vi "Disable_Enable.vi"(6 "menu reference":refnum<k9>, 7 "Disabled":T2(ring)=enum."Disabled and Grayed Out", 8 "error in (no error)":errorcluster, 10 "Command":T1=enum."INIT", 11 "EpiWrapper in":refnum<class "EpiWrapper.lvclass">) -> (0 "error out":errorcluster, 3 "EpiWrapper out":refnum<class "EpiWrapper.lvclass">)   [LabVIEW 2012, in "EpiWrapper.lvclass"]
uses:
  EpiWrapper.lvclass
  Controls/Command_Enum.ctl
  Controls/Control_Selector.ctl
  Controls/Input_Selector.ctl
  EpiWrapper.lvclass/EpiWrapper.ctl
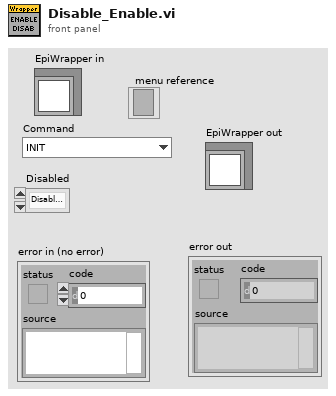
[diagram p1: front panel]
types:
  T1 = typedef "Command_Enum.ctl" = enum16{"SPECTRUMCAPTURE", "INSITUMEASURE", "RESETCONFIG", "OPENCONFIG", "RESET", "INIT", "LOAD", "MEASURE", "NEW", "SAVE", "UPDATE_INT", "SWAP_MODE", "UPDATE_ACQ", "MARK_MAP_SELECT", "MARK_MAP", "EXIT", "CANCEL"}
  T2 = enum8{"Enabled", "Disabled", "Disabled and Grayed Out"}
  T3 = typedef "Input_Selector.ctl" = enum16{"Wafer ID", "Test", "New", "Save", "Load", "Cancel"}
  T4 = typedef "Control_Selector.ctl" = enum16{"Plot", "Pass", "Fail", "Measure", "Area", "TestData", "Pad"}
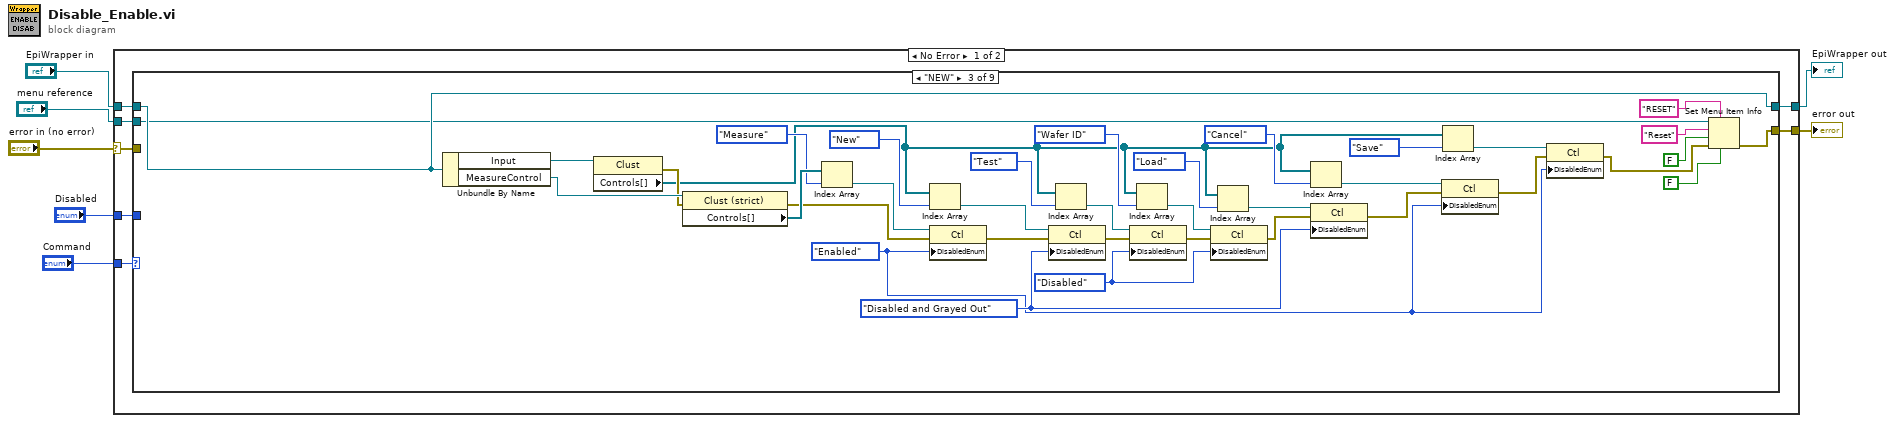
[diagram p0: block diagram]
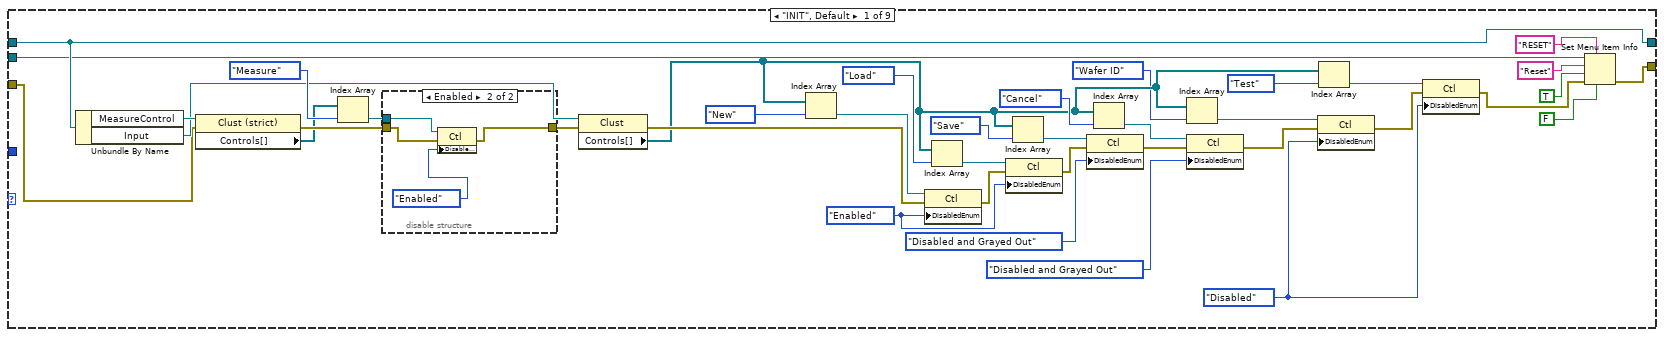
[diagram p2: hidden frame]
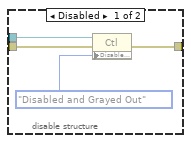
[diagram p3: hidden frame]
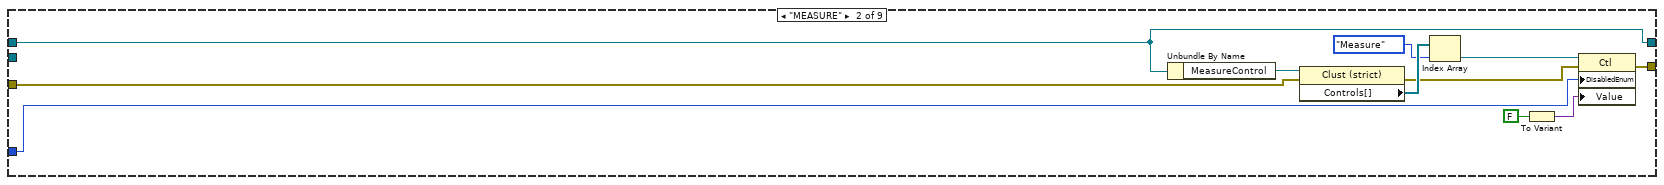
[diagram p4: hidden frame]
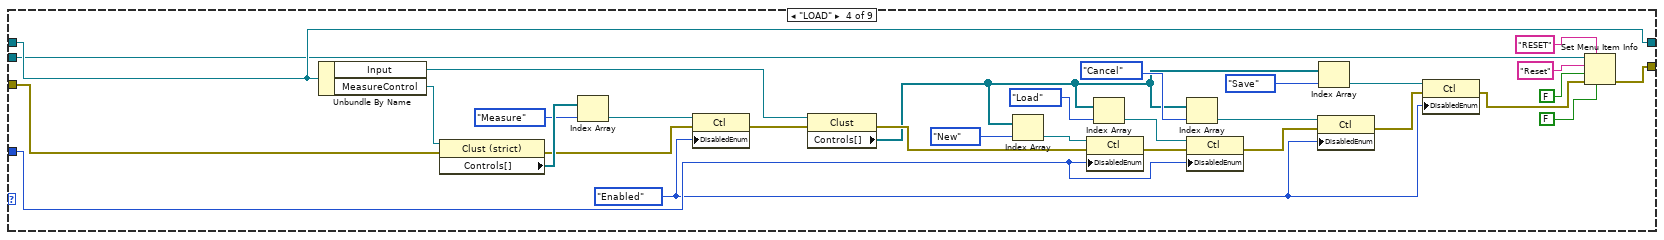
[diagram p5: hidden frame]
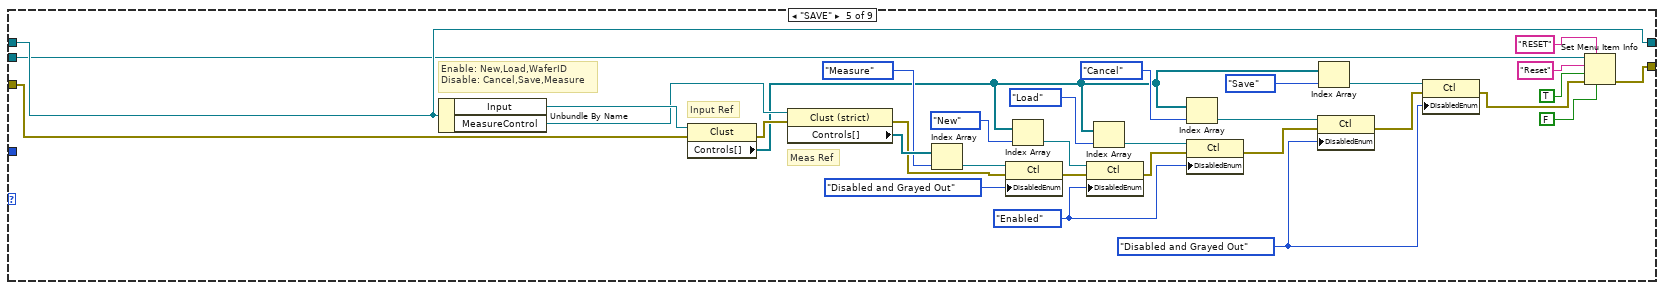
[diagram p6: hidden frame]
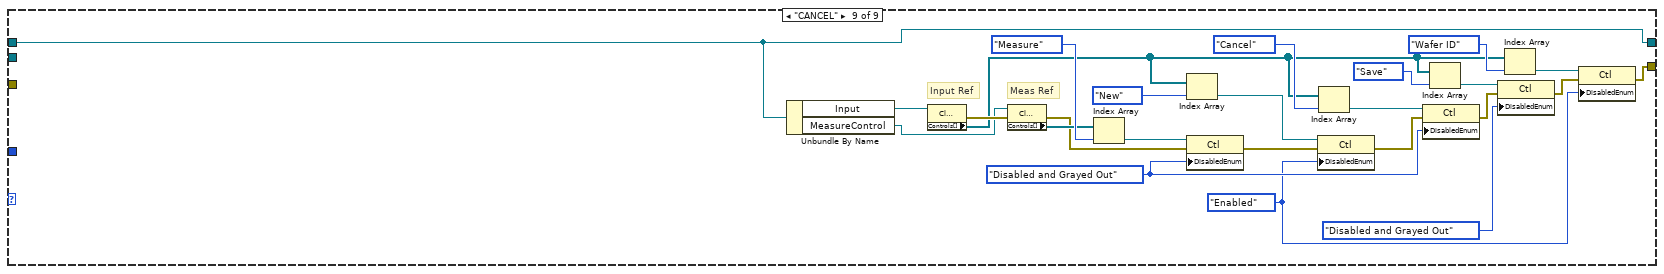
[diagram p10: hidden frame]
diagram:
  n1 = case shown="No Error" "error in (no error)" {
    selector: "error in (no error)" -> [w10 w205]
    tunnel: [w11 w205] -> w6
    tunnel: [w9 w204] -> w4
    tunnel: "EpiWrapper in" -> [w13 w204]
    tunnel: "Command" -> [w14 _]
    tunnel: "Disabled" -> [w12 _]
    tunnel: "menu reference" -> [w8 _]
    frame No Error {
      n2 = case shown="\"NEW\"" w14 {
        tunnel: w13 -> [w44 w64 w96 w132 w154 w174 w176 w178 w191]
        tunnel: w12 -> [_ w65 _ w135 _ _ _ _ _]
        tunnel: [w17 w66 w73 w112 w147 w173 w175 w177 w179] -> w11
        tunnel: w10 -> [w15 w68 _ w130 w153 w173 w175 w177 _]
        tunnel: [w44 w64 w96 w132 w154 w174 w176 w178 w191] -> w9
        tunnel: w8 -> [w16 _ w75 w110 w145 _ _ _ _]
        frame "INIT", Default {
          w23 = T2."Disabled" ("Disabled")
          w33 = T2."Enabled" ("Disabled")
          n3 = Unbundle By Name(w44) -> ("MeasureControl"=w47:refnum<vi>, "Input"=w46:refnum<vi>)
          n4 = property class="Clust (strict)"(reference=w47, error in=w15) -> (error out=w50:errorcluster, "Controls[]"=w45:refnum<vi>[])  [unwired: 1 out]
          n5 = Index Array(array=w45, index=Control_Selector."Measure" ("Control_Selector")) -> (element=w49:refnum<vi>)
          n6 = disable-structure shown="Enabled" {
            disable-tunnel: [w57 w59] -> w53
            disable-tunnel: w50 -> [w56 w60]
            disable-tunnel: w49 -> [w55 w61]
            frame Disabled {
              n7 = property class="Ctl"(reference=w55, error in=w56, "DisabledEnum"=T2."Disabled and Grayed Out" ("Disabled")) -> (error out=w57:errorcluster)  [unwired: 1 out]
            }
            frame Enabled {
              n8 = property class="Ctl"(reference=w61, error in=w60, "DisabledEnum"=T2."Enabled" ("Disabled")) -> (error out=w59:errorcluster)  [unwired: 1 out]
            }
          }
          n9 = property class="Clust"(reference=w46, error in=w53) -> (error out=w37:errorcluster, "Controls[]"=w30:refnum<vi>[])  [unwired: 1 out]
          n10 = Index Array(array=w30, index=Input_Selector."New" ("InputSelector")) -> (element=w51:refnum<vi>)
          n11 = property class="Ctl"(reference=w51, error in=w37, "DisabledEnum"=w33) -> (error out=w32:errorcluster)  [unwired: 1 out]
          n12 = Index Array(array=w30, index=Input_Selector."Load" ("InputSelector")) -> (element=w34:refnum<vi>)
          n13 = property class="Ctl"(reference=w34, error in=w32, "DisabledEnum"=w33) -> (error out=w31:errorcluster)  [unwired: 1 out]
          n14 = Index Array(array=w30, index=Input_Selector."Save" ("InputSelector")) -> (element=w39:refnum<vi>)
          n15 = property class="Ctl"(reference=w39, error in=w31, "DisabledEnum"=T2."Disabled and Grayed Out" ("Disabled")) -> (error out=w36:errorcluster)  [unwired: 1 out]
          n16 = Index Array(array=w30, index=Input_Selector."Cancel" ("InputSelector")) -> (element=w38:refnum<vi>)
          n17 = Index Array(array=w30, index=Input_Selector."Wafer ID" ("InputSelector")) -> (element=w25:refnum<vi>)
          n18 = property class="Ctl"(reference=w38, error in=w36, "DisabledEnum"=T2."Disabled and Grayed Out" ("Disabled")) -> (error out=w26:errorcluster)  [unwired: 1 out]
          n19 = property class="Ctl"(reference=w25, error in=w26, "DisabledEnum"=w23) -> (error out=w27:errorcluster)  [unwired: 1 out]
          n20 = Index Array(array=w30, index=Input_Selector."Test" ("InputSelector")) -> (element=w24:refnum<vi>)
          n21 = property class="Ctl"(reference=w24, error in=w27, "DisabledEnum"=w23) -> (error out=w18:errorcluster)  [unwired: 1 out]
          n22 = Set Menu Item Info(6:FALSE ("checked"), 7:"RESET" ("item name"), 8:w18, 9:TRUE ("enabled"), 10:"Reset" ("item name"), 11:w16) -> (0:w17:errorcluster)  [unwired: 1 in, 1 out]
        }
        frame "MEASURE" {
          n23 = Unbundle By Name(w64) -> ("MeasureControl"=w71:refnum<vi>)
          n24 = property class="Clust (strict)"(reference=w71, error in=w68) -> (error out=w67:errorcluster, "Controls[]"=w72:refnum<vi>[])  [unwired: 1 out]
          n25 = Index Array(array=w72, index=Control_Selector."Measure" ("Control_Selector")) -> (element=w69:refnum<vi>)
          n26 = To Variant(anything=FALSE) -> (Variant=w62:variant)
          n27 = property class="Ctl"(reference=w69, error in=w67, "DisabledEnum"=w65, "Value"=w62) -> (error out=w66:errorcluster)  [unwired: 1 out]
        }
        frame "NEW" {
          w85 = T2."Disabled" ("Disabled")
          w88 = T2."Disabled and Grayed Out" ("Disabled")
          w81 = T2."Enabled" ("Disabled")
          n28 = Unbundle By Name(w96) -> ("Input"=w108:refnum<vi>, "MeasureControl"=w106:refnum<vi>)
          n29 = property class="Clust"(reference=w108) -> (error out=w105:errorcluster, "Controls[]"=w83:refnum<vi>[])  [unwired: 1 in, 1 out]
          n30 = property class="Clust (strict)"(reference=w106, error in=w105) -> (error out=w101:errorcluster, "Controls[]"=w104:refnum<vi>[])  [unwired: 1 out]
          n31 = Index Array(array=w104, index=Control_Selector."Measure" ("Control_Selector")) -> (element=w102:refnum<vi>)
          n32 = Index Array(array=w83, index=Input_Selector."New" ("InputSelector")) -> (element=w109:refnum<vi>)
          n33 = property class="Ctl"(reference=w102, error in=w101, "DisabledEnum"=w81) -> (error out=w100:errorcluster)  [unwired: 1 out]
          n34 = property class="Ctl"(reference=w109, error in=w100, "DisabledEnum"=w88) -> (error out=w93:errorcluster)  [unwired: 1 out]
          n35 = Index Array(array=w83, index=Input_Selector."Test" ("InputSelector")) -> (element=w94:refnum<vi>)
          n36 = property class="Ctl"(reference=w94, error in=w93, "DisabledEnum"=w85) -> (error out=w92:errorcluster)  [unwired: 1 out]
          n37 = Index Array(array=w83, index=Input_Selector."Wafer ID" ("InputSelector")) -> (element=w98:refnum<vi>)
          n38 = property class="Ctl"(reference=w98, error in=w92, "DisabledEnum"=w85) -> (error out=w89:errorcluster)  [unwired: 1 out]
          n39 = Index Array(array=w83, index=Input_Selector."Load" ("InputSelector")) -> (element=w90:refnum<vi>)
          n40 = Index Array(array=w83, index=Input_Selector."Cancel" ("InputSelector")) -> (element=w87:refnum<vi>)
          n41 = property class="Ctl"(reference=w90, error in=w89, "DisabledEnum"=w88) -> (error out=w86:errorcluster)  [unwired: 1 out]
          n42 = property class="Ctl"(reference=w87, error in=w86, "DisabledEnum"=w81) -> (error out=w80:errorcluster)  [unwired: 1 out]
          n43 = Index Array(array=w83, index=Input_Selector."Save" ("InputSelector")) -> (element=w84:refnum<vi>)
          n44 = property class="Ctl"(reference=w84, error in=w80, "DisabledEnum"=w81) -> (error out=w74:errorcluster)  [unwired: 1 out]
          n45 = Set Menu Item Info(6:FALSE ("checked"), 7:"RESET" ("item name"), 8:w74, 9:FALSE ("enabled"), 10:"Reset" ("item name"), 11:w75) -> (0:w73:errorcluster)  [unwired: 1 in, 1 out]
        }
        frame "LOAD" {
          w117 = T2."Enabled" ("Disabled")
          n46 = Unbundle By Name(w132) -> ("Input"=w139:refnum<vi>, "MeasureControl"=w131:refnum<vi>)
          n47 = property class="Clust (strict)"(reference=w131, error in=w130) -> (error out=w126:errorcluster, "Controls[]"=w129:refnum<vi>[])  [unwired: 1 out]
          n48 = Index Array(array=w129, index=Control_Selector."Measure" ("Control_Selector")) -> (element=w127:refnum<vi>)
          n49 = property class="Ctl"(reference=w127, error in=w126, "DisabledEnum"=w117) -> (error out=w125:errorcluster)  [unwired: 1 out]
          n50 = property class="Clust"(reference=w139, error in=w125) -> (error out=w133:errorcluster, "Controls[]"=w120:refnum<vi>[])  [unwired: 1 out]
          n51 = Index Array(array=w120, index=Input_Selector."New" ("InputSelector")) -> (element=w140:refnum<vi>)
          n52 = property class="Ctl"(reference=w140, error in=w133, "DisabledEnum"=w135) -> (error out=w134:errorcluster)  [unwired: 1 out]
          n53 = Index Array(array=w120, index=Input_Selector."Load" ("InputSelector")) -> (element=w136:refnum<vi>)
          n54 = Index Array(array=w120, index=Input_Selector."Cancel" ("InputSelector")) -> (element=w123:refnum<vi>)
          n55 = property class="Ctl"(reference=w136, error in=w134, "DisabledEnum"=w135) -> (error out=w122:errorcluster)  [unwired: 1 out]
          n56 = property class="Ctl"(reference=w123, error in=w122, "DisabledEnum"=w117) -> (error out=w121:errorcluster)  [unwired: 1 out]
          n57 = Index Array(array=w120, index=Input_Selector."Save" ("InputSelector")) -> (element=w118:refnum<vi>)
          n58 = property class="Ctl"(reference=w118, error in=w121, "DisabledEnum"=w117) -> (error out=w111:errorcluster)  [unwired: 1 out]
          n59 = Set Menu Item Info(6:FALSE ("checked"), 7:"RESET" ("item name"), 8:w111, 9:FALSE ("enabled"), 10:"Reset" ("item name"), 11:w110) -> (0:w112:errorcluster)  [unwired: 1 in, 1 out]
        }
        frame "SAVE" {
          w156 = T2."Enabled" ("Disabled")
          w148 = T2."Disabled and Grayed Out" ("Disabled")
          # "Enable: New,Load,WaferID\nDisable: Cancel,Save,Measure"
          # "Input Ref"
          # "Meas Ref"
          n60 = Unbundle By Name(w154) -> ("Input"=w171:refnum<vi>, "MeasureControl"=w169:refnum<vi>)
          n61 = property class="Clust"(reference=w171, error in=w153) -> (error out=w168:errorcluster, "Controls[]"=w152:refnum<vi>[])  [unwired: 1 out]
          n62 = property class="Clust (strict)"(reference=w169, error in=w168) -> (error out=w164:errorcluster, "Controls[]"=w167:refnum<vi>[])  [unwired: 1 out]
          n63 = Index Array(array=w167, index=Control_Selector."Measure" ("Control_Selector")) -> (element=w165:refnum<vi>)
          n64 = property class="Ctl"(reference=w165, error in=w164, "DisabledEnum"=T2."Disabled and Grayed Out" ("Disabled")) -> (error out=w163:errorcluster)  [unwired: 1 out]
          n65 = Index Array(array=w152, index=Input_Selector."New" ("InputSelector")) -> (element=w172:refnum<vi>)
          n66 = property class="Ctl"(reference=w172, error in=w163, "DisabledEnum"=w156) -> (error out=w155:errorcluster)  [unwired: 1 out]
          n67 = Index Array(array=w152, index=Input_Selector."Load" ("InputSelector")) -> (element=w161:refnum<vi>)
          n68 = Index Array(array=w152, index=Input_Selector."Cancel" ("InputSelector")) -> (element=w159:refnum<vi>)
          n69 = property class="Ctl"(reference=w161, error in=w155, "DisabledEnum"=w156) -> (error out=w158:errorcluster)  [unwired: 1 out]
          n70 = property class="Ctl"(reference=w159, error in=w158, "DisabledEnum"=w148) -> (error out=w149:errorcluster)  [unwired: 1 out]
          n71 = Index Array(array=w152, index=Input_Selector."Save" ("InputSelector")) -> (element=w150:refnum<vi>)
          n72 = property class="Ctl"(reference=w150, error in=w149, "DisabledEnum"=w148) -> (error out=w146:errorcluster)  [unwired: 1 out]
          n73 = Set Menu Item Info(6:FALSE ("checked"), 7:"RESET" ("item name"), 8:w146, 9:TRUE ("enabled"), 10:"Reset" ("item name"), 11:w145) -> (0:w147:errorcluster)  [unwired: 1 in, 1 out]
        }
        frame "SWAP_MODE" {
        }
        frame "UPDATE_ACQ" {
        }
        frame "EXIT" {
        }
        frame "CANCEL" {
          w180 = T2."Enabled" ("Disabled")
          w187 = T2."Disabled and Grayed Out" ("Disabled")
          # "Meas Ref"
          # "Input Ref"
          n74 = Unbundle By Name(w191) -> ("Input"=w203:refnum<vi>, "MeasureControl"=w196:refnum<vi>)
          n75 = property class="Clust"(reference=w203) -> (error out=w197:errorcluster, "Controls[]"=w181:refnum<vi>[])  [unwired: 1 in, 1 out]
          n76 = property class="Clust (strict)"(reference=w196, error in=w197) -> (error out=w194:errorcluster, "Controls[]"=w195:refnum<vi>[])  [unwired: 1 out]
          n77 = Index Array(array=w195, index=Control_Selector."Measure" ("Control_Selector")) -> (element=w193:refnum<vi>)
          n78 = Index Array(array=w181, index=Input_Selector."New" ("InputSelector")) -> (element=w190:refnum<vi>)
          n79 = property class="Ctl"(reference=w193, error in=w194, "DisabledEnum"=w187) -> (error out=w192:errorcluster)  [unwired: 1 out]
          n80 = property class="Ctl"(reference=w190, error in=w192, "DisabledEnum"=w180) -> (error out=w199:errorcluster)  [unwired: 1 out]
          n81 = Index Array(array=w181, index=Input_Selector."Cancel" ("InputSelector")) -> (element=w188:refnum<vi>)
          n82 = property class="Ctl"(reference=w188, error in=w199, "DisabledEnum"=w187) -> (error out=w184:errorcluster)  [unwired: 1 out]
          n83 = Index Array(array=w181, index=Input_Selector."Save" ("InputSelector")) -> (element=w186:refnum<vi>)
          n84 = property class="Ctl"(reference=w186, error in=w184, "DisabledEnum"=T2."Disabled and Grayed Out" ("Disabled")) -> (error out=w183:errorcluster)  [unwired: 1 out]
          n85 = Index Array(array=w181, index=Input_Selector."Wafer ID" ("InputSelector")) -> (element=w182:refnum<vi>)
          n86 = property class="Ctl"(reference=w182, error in=w183, "DisabledEnum"=w180) -> (error out=w179:errorcluster)  [unwired: 1 out]
        }
      }
    }
    frame Error {
    }
  }
  "error out" <- w6
  "EpiWrapper out" <- w4
